vi "Write Report Folder.vi"(8 "error in (no error)":errorcluster, 10 "Report Folder":path, 11 "Project Action in":refnum<class "Project Action.lvclass">) -> (0 "error out":errorcluster, 3 "Project Action out":refnum<class "Project Action.lvclass">)   [LabVIEW 2020, in "ProjectBuilder.lvlib" / "Project Action.lvclass"]
uses:
  Project Action.lvclass
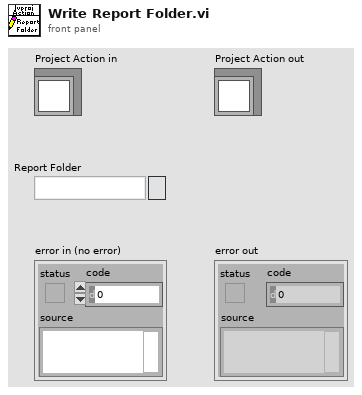
[diagram p1: front panel]
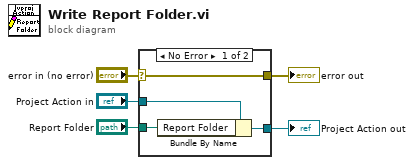
[diagram p0: block diagram]
diagram:
  n1 = case shown="No Error" "error in (no error)" {
    selector: "error in (no error)" -> [w9 w10]
    tunnel: [w9 w10] -> w4
    tunnel: [w7 w11] -> w2
    tunnel: "Project Action in" -> [w8 w11]
    tunnel: "Report Folder" -> [w6 _]
    frame No Error {
      n2 = Bundle By Name(cluster=w8, "Report Folder"=w6) -> (w7:refnum<class "Project Action.lvclass">)
    }
    frame Error {
    }
  }
  "error out" <- w4
  "Project Action out" <- w2
